vi "ATEPanelUltraSafe.vi"(2 "error in (no error)":errorcluster) -> (0 "Error out":errorcluster)   [LabVIEW 2009]
doc: "Place ATE plate switches and attenuators in ultra safe states (work in progress)"
panel:
  # "UltraSafe leaves tx disabled"
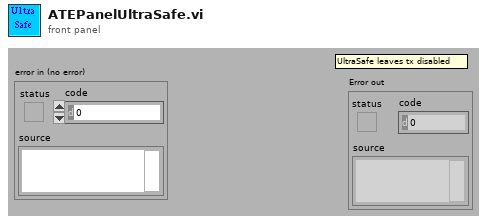
[diagram p1: front panel]
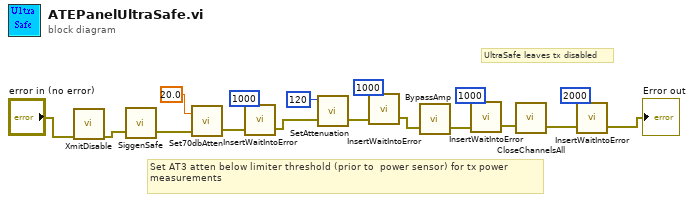
[diagram p0: block diagram]
diagram:
  # "UltraSafe leaves tx disabled"
  # "Set AT3 atten below limiter threshold (prior to  power sensor) for tx power measurements"
  n1 = call "XmitDisable.vi"("error in (no error)"="error in (no error)") -> ("error out"=w14:errorcluster)  [unwired: 1 in, 5 out]
  n2 = call "SiggenSafe.vi"("error in (no error)"=w14) -> ("error out"=w12:errorcluster)  [unwired: 2 in]
  n3 = call "Set70dbAtten.vi"("error in (no error)"=w12, "Attenuation (dB)"=20.0) -> ("error out"=w6:errorcluster)  [unwired: 1 in]
  n4 = call "InsertWaitIntoError.vi"("error in (no error)"=w6, "Wait (msecs)"=1000) -> ("error out"=w5:errorcluster)  [unwired: 1 in]
  n5 = call "SetAttenuation.vi"("error in (no error)"=w5, "Attenuation (dB)"=120) -> ("error out"=w4:errorcluster)  [unwired: 1 in]
  n6 = call "InsertWaitIntoError.vi"("error in (no error)"=w4, "Wait (msecs)"=1000) -> ("error out"=w3:errorcluster)  [unwired: 1 in]
  n7 = call "BypassAmp.vi"("error in (no error)"=w3) -> ("error out"=w2:errorcluster)  [unwired: 2 in]
  n8 = call "InsertWaitIntoError.vi"("error in (no error)"=w2, "Wait (msecs)"=1000) -> ("error out"=w1:errorcluster)  [unwired: 1 in]
  n9 = call "CloseChannelsAll.vi"("error in (no error)"=w1) -> ("error out"=w15:errorcluster)  [unwired: 2 in]
  n10 = call "InsertWaitIntoError.vi"("error in (no error)"=w15, "Wait (msecs)"=2000) -> ("error out"=→"Error out":errorcluster)  [unwired: 1 in]
